vi "Test simple.vi"() -> ()   [LabVIEW 2017]
uses:
  Quality.ctl
  Filter.ctl
  Range.ctl
panel:
  out "Range out":T1 items=["Auto range", "2nA", "20nA", "200nA", "2uA", "20uA", "200uA", "2mA"]
  in  "Range":T1 items=["Auto range", "2nA", "20nA", "200nA", "2uA", "20uA", "200uA", "2mA"]
  out "Filter out":T2 items=["No filter", "2", "4", "8", "16", "32", "64"]
  in  "Filter":T2 items=["No filter"=0, "2"=2, "4"=4, "8"=8, "16"=16, "32"=32, "64"=64]
  out "Quality":T3
  out "Value, nA":dbl
  in  "VISA resource name":refnum<visa-resource-name>="COM4"
  in  "BtnMeasure":bool
  in  "BtnStop":bool
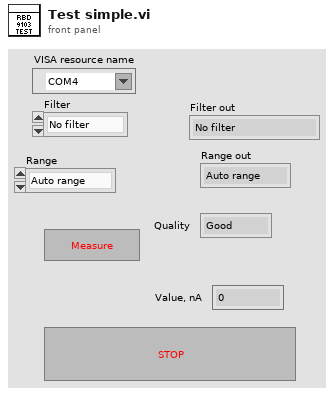
[diagram p1: front panel]
types:
  T1 = typedef "Range.ctl" = u16
  T2 = typedef "Filter.ctl" = u16
  T3 = typedef "Quality.ctl" = enum16{"Good", "Unstable", "Under", "Over"}
  T4 = typedef "RBD9103.ctl" = cluster{"Serial port sem":T5, "Serial port handle":refnum<visa-resource-name>, "Controller #":u8, "Firmware":string, "Device ID":i32, "UI events":T6}
  T5 = typedef "Semaphore RefNum" = refnum<k1>
  T6 = typedef "GenericEvent.ctl" = refnum<user-event>
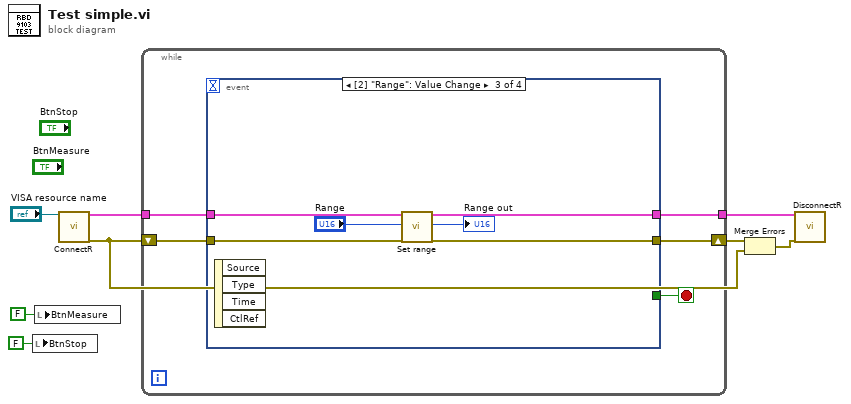
[diagram p0: block diagram]
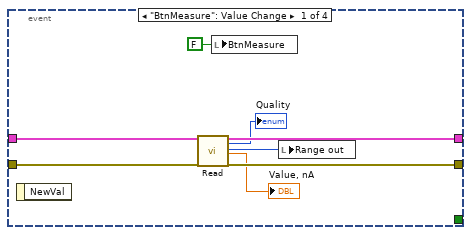
[diagram p2: hidden frame]
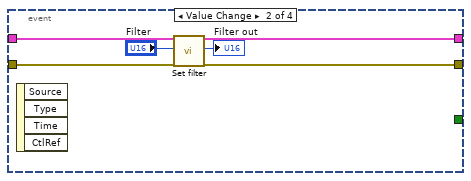
[diagram p3: hidden frame]
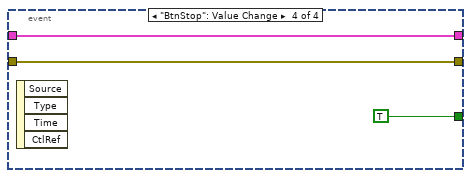
[diagram p4: hidden frame]
diagram:
  n1 = local write "BtnStop"(FALSE ("BtnStop")) -> ()
  n2 = local write "BtnMeasure"(FALSE ("BtnMeasure")) -> ()
  n3 = call "ConnectR.vi"("VISA resource name"="VISA resource name") -> ("RBD9103"=w5:T4, "error out"=w2:errorcluster)  [unwired: 17 in]
  n4 = while {
    tunnel: w5 -> [w13]
    tunnel: [w9] -> w4
    shift-right: [w10] -> w3
    shift-left: w2 -> [w12]
    stop <- w11 stop-if-true
    n5 = event shown="[2] \"Range\": Value Change" {
      selector: _ -> [_ _ _ _]
      dyn-events: _ -> [_ _ _ _]
      timeout: _ -> [_ _ _ _]
      tunnel: w13 -> [w18 w25 w32 w34]
      tunnel: w12 -> [w17 w26 w33 w35]
      tunnel: [_ _ _ TRUE] -> w11
      tunnel: [w20 w23 w30 w35] -> w10
      tunnel: [w19 w24 w31 w34] -> w9
      event "BtnMeasure": Value Change {
        n6 = event-data() -> ()  [unwired: 1 in, 1 out]
        n7 = call "Read.vi"("RBD9103"=w18, "error in"=w17) -> ("RBD9103 out"=w19:T4, "Quality"=→"Quality":T3, "Range out"=w14:T1, "Value, nA"=→"Value, nA":dbl, "error out"=w20:errorcluster)  [unwired: 12 in, 1 out]
        n8 = local write "BtnMeasure"(FALSE ("BtnMeasure")) -> ()
        n9 = local write "Range out"(w14) -> ()
      }
      event Value Change {
        n10 = event-data() -> ()  [unwired: 1 in, 4 out]
        n11 = call "Set filter.vi"("RBD9103"=w25, "Filter"="Filter", "error in"=w26) -> ("RBD9103 out"=w24:T4, "Filter"=→"Filter out":T2, "error out"=w23:errorcluster)  [unwired: 14 in]
      }
      event Value Change {
        n12 = event-data() -> ()  [unwired: 1 in, 4 out]
        n13 = call "Set range.vi"("RBD9103"=w32, "Range"="Range", "error in"=w33) -> ("RBD9103 out"=w31:T4, "Range out"=→"Range out":T1, "error out"=w30:errorcluster)  [unwired: 14 in]
      }
      event "BtnStop": Value Change {
        n14 = event-data() -> ()  [unwired: 1 in, 4 out]
      }
    }
  }
  n15 = Merge Errors(w3, w2) -> (w1:errorcluster)
  n16 = call "DisconnectR.vi"("RBD9103"=w4, "error in"=w1) -> ()  [unwired: 17 in, 1 out]
